vi "Encoder Distance.vi"() -> ()   [LabVIEW 2016]
panel:
  out "W)(33L D1574NC3":dbl
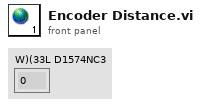
[diagram p1: front panel]
diagram:
